vi "multicolumn_pass.vi"(0 "LstBox Refnum":refnum<vi>, 1 "Frekanslar":dbl[](array[numeric]), 2 "interrupt(F)":bool, 5 "MCListbox Refnum":refnum<vi>, 7 "Denge Kosulu x2_y2":dbl[][](array[numeric]), 9 "Denge Kosulu x1_x2":dbl[][](array[numeric]), 11 "Denge Kosulu y1_y2":dbl[][](array[numeric]), 12 "frekans index":dbl, 13 "F values array":dbl[][](array[numeric])) -> (4 "Output Denge Kosulu x2_y2":dbl[][](array[numeric]), 6 "Output Denge Kosulu x1_x2":dbl[][](array[numeric]), 8 "Outpu Denge Kosulu y1_y2":dbl[][](array[numeric]))   [LabVIEW 2014]
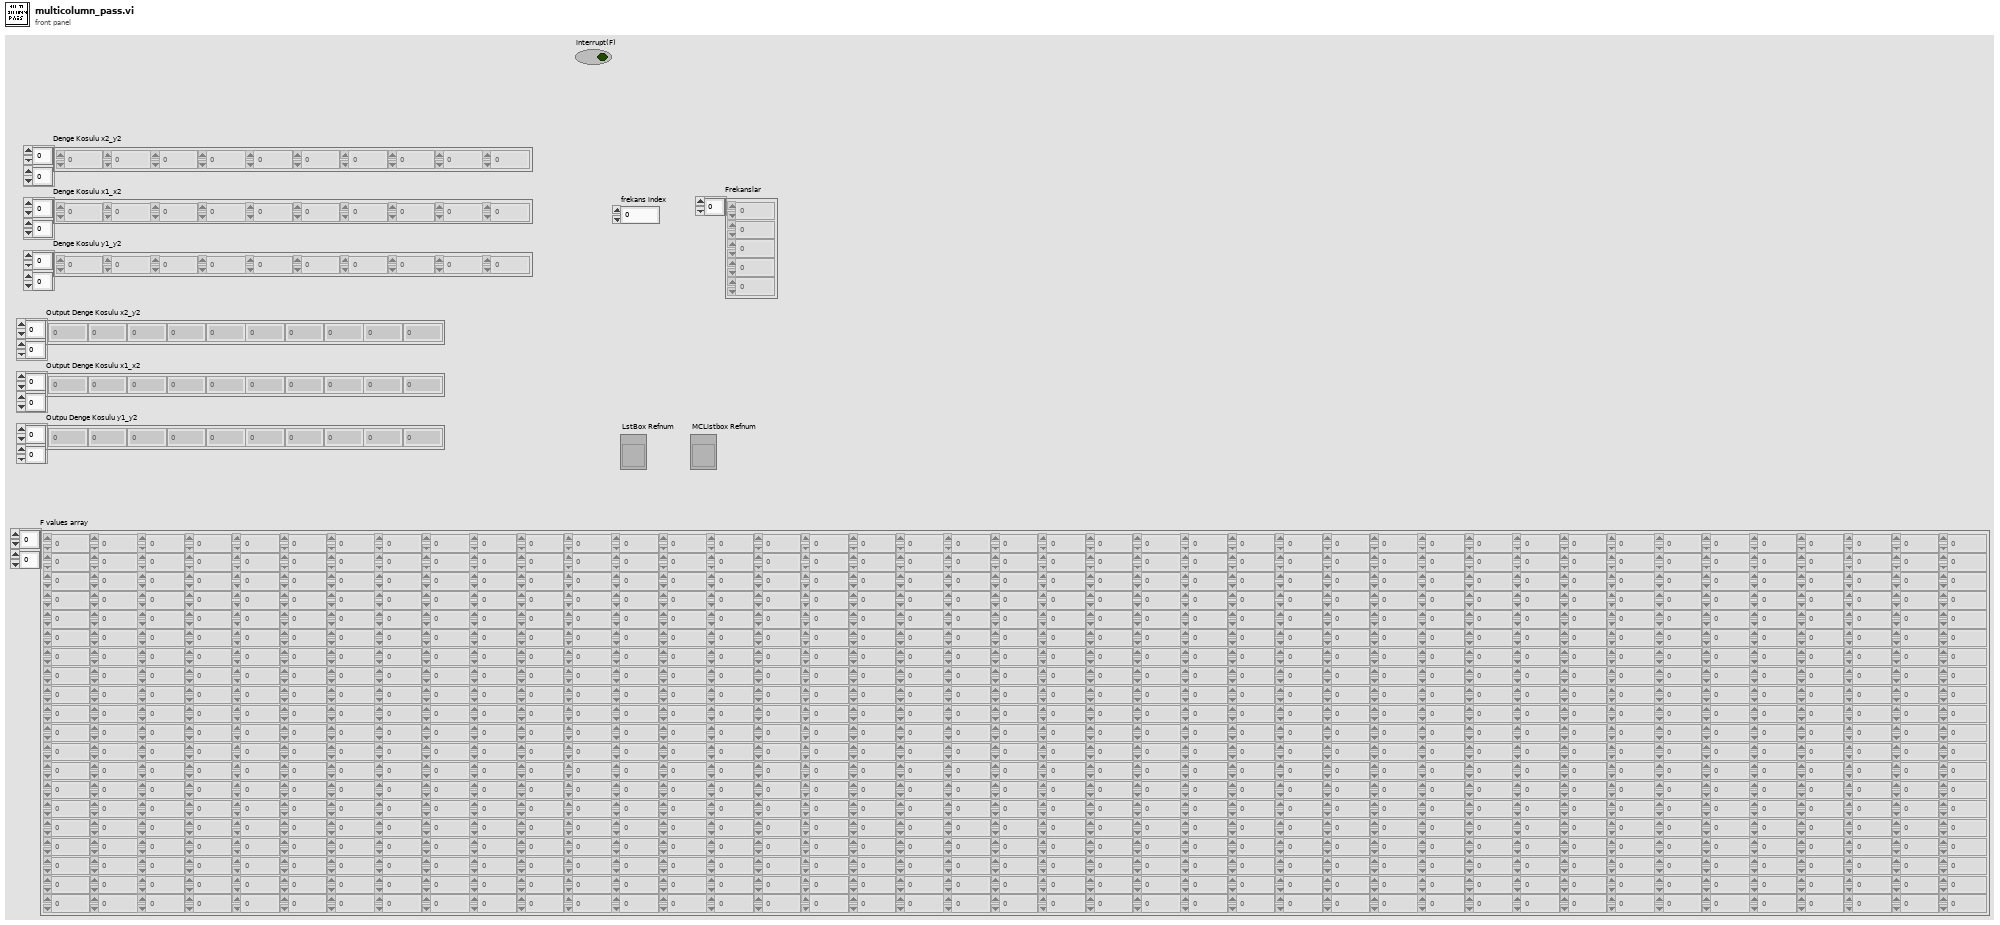
[diagram p1: front panel]
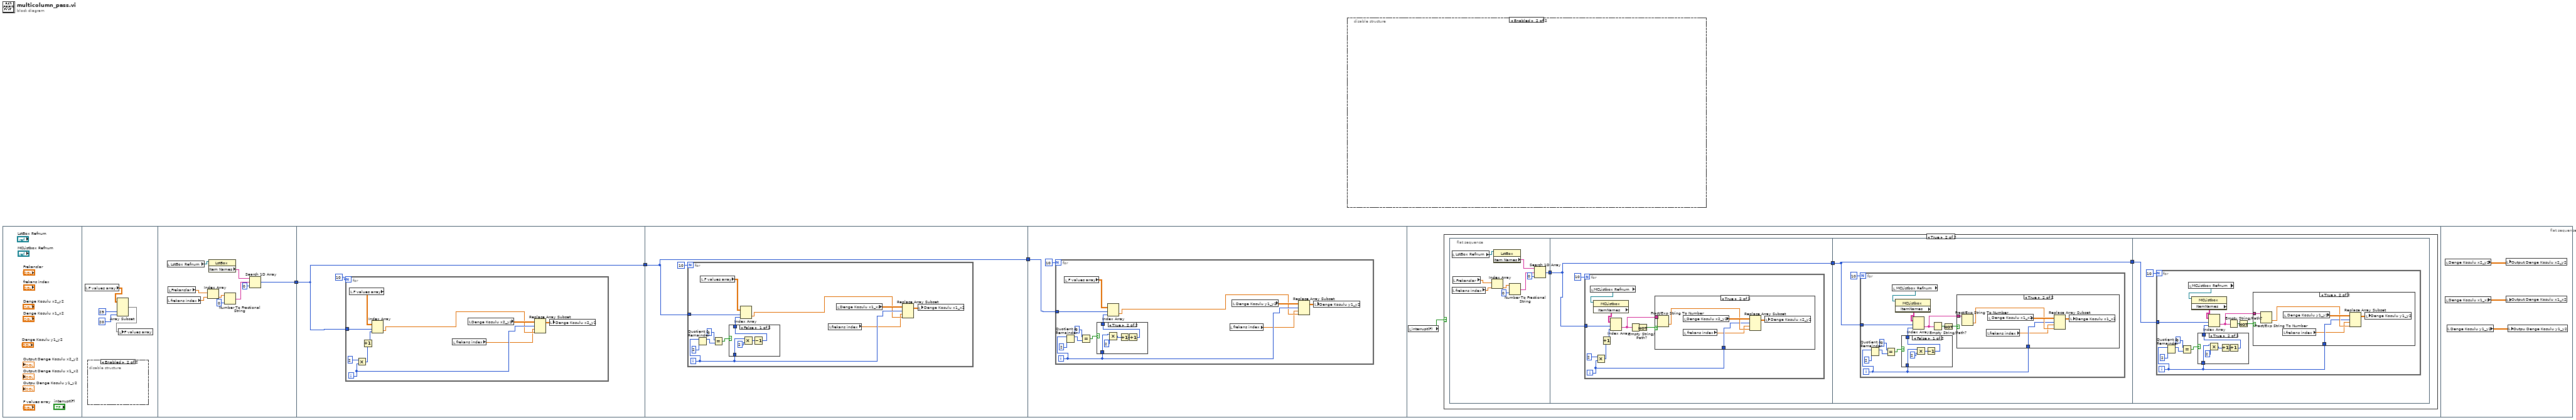
[diagram p0: block diagram]
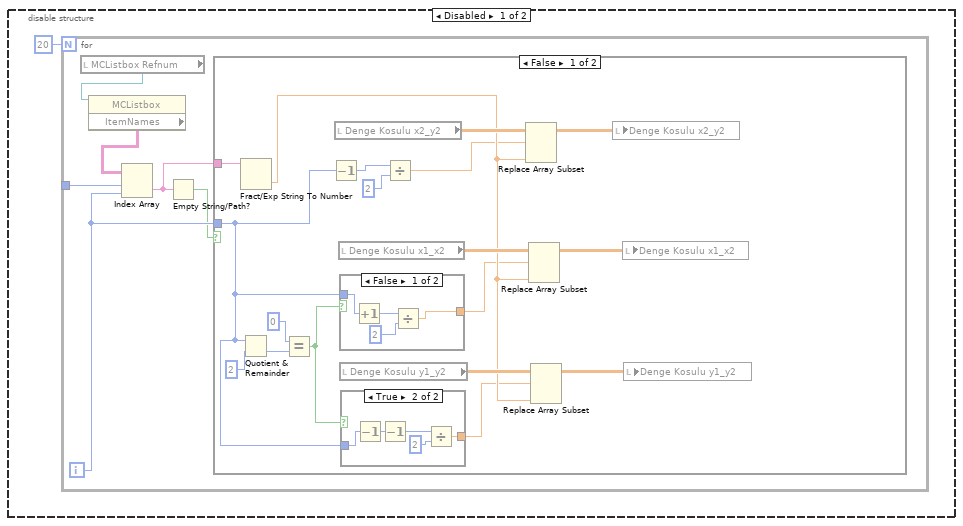
[diagram p2: hidden frame]
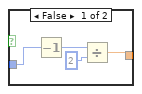
[diagram p3: hidden frame]
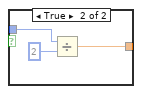
[diagram p4: hidden frame]
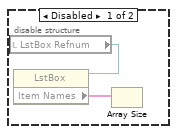
[diagram p6: hidden frame]
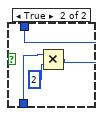
[diagram p7: hidden frame]
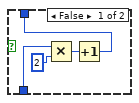
[diagram p8: hidden frame]
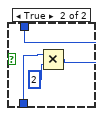
[diagram p11: hidden frame]
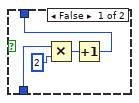
[diagram p13: hidden frame]
diagram:
  n1 = flat-sequence {
    tunnel: [w11] -> w3
    tunnel: w3 -> [w20]
    tunnel: [w20] -> w2
    tunnel: w2 -> [w32]
    tunnel: [w32] -> w1
    tunnel: w1 -> [w53]
    frame #0 {
    }
    frame #1 {
      n2 = local read "F values array"() -> (w7:dbl[][])
      n3 = disable-structure shown="Enabled" {
        frame Disabled {
          n4 = local read "LstBox Refnum"() -> (w10:refnum<vi>)
          n5 = property class="LstBox"(reference=w10) -> ("Item Names"=w9:string[])  [unwired: 1 in, 2 out]
          n6 = Array Size(array=w9) -> (size(s)=w8:i32)
        }
        frame Enabled {
        }
      }
      n7 = Array Subset(array=w7, index (col)=29 ("index"), length (col)=20 ("length")) -> (w4:dbl[][])  [unwired: 2 in]
      n8 = local write "F values array"(w4) -> ()
    }
    frame #2 {
      n9 = local read "LstBox Refnum"() -> (w19:refnum<vi>)
      n10 = local read "frekans index"() -> (w17:dbl)
      n11 = local read "Frekanslar"() -> (w18:dbl[])
      n12 = Index Array(array=w18, index=w17) -> (element=w16:dbl)
      n13 = property class="LstBox"(reference=w19) -> ("Item Names"=w15:string[])  [unwired: 1 in, 2 out]
      n14 = Number To Fractional String(number=w16, precision (6)=i16 0) -> (F-format string=w14:string)  [unwired: 2 in]
      n15 = Search 1D Array(1D array=w15, element=w14, start index (0)=0) -> (index of element=w11:i32)
    }
    frame #3 {
      n16 = for {
        N: 10 -> [_]
        tunnel: w20 -> [w27]
        i -> [w28]
        n17 = local read "F values array"() -> (w26:dbl[][])
        n18 = Multiply(x=2, y=w28) -> (x*y=w30:i32)
        n19 = Increment(x=w30) -> (x+1=w29:i32)
        n20 = Index Array(array=w26, index (row)=w27, index (col)=w29) -> (element=w23:dbl)
        n21 = local read "frekans index"() -> (w22:dbl)
        n22 = local read "Denge Kosulu x2_y2"() -> (w24:dbl[][])
        n23 = Replace Array Subset(array=w24, new element=w23, index (row)=w28, index (col)=w22) -> (w25:dbl[][])
        n24 = local write "Denge Kosulu x2_y2"(w25) -> ()
      }
    }
    frame #4 {
      n25 = for {
        N: 10 -> [_]
        tunnel: w32 -> [w40]
        i -> [w42]
        n26 = Quotient & Remainder(x=w42, y=2) -> (x-y*floor(x/y)=w39:i32)  [unwired: 1 out]
        n27 = local read "F values array"() -> (w38:dbl[][])
        n28 = Equal?(x=0, y=w39) -> (x = y?=w43:bool)
        n29 = case shown="False" w43 {
          tunnel: w42 -> [w49 w52]
          tunnel: [w46 w50] -> w41
          frame False {
            n30 = Multiply(x=w49, y=2) -> (x*y=w47:i32)
            n31 = Decrement(x=w47) -> (x-1=w46:i32)
          }
          frame True {
            n32 = Multiply(x=w52, y=2) -> (x*y=w50:i32)
          }
        }
        n33 = Index Array(array=w38, index (row)=w40, index (col)=w41) -> (element=w35:dbl)
        n34 = local read "frekans index"() -> (w34:dbl)
        n35 = local read "Denge Kosulu x1_x2"() -> (w36:dbl[][])
        n36 = Replace Array Subset(array=w36, new element=w35, index (row)=w42, index (col)=w34) -> (w37:dbl[][])
        n37 = local write "Denge Kosulu x1_x2"(w37) -> ()
      }
    }
    frame #5 {
      n38 = for {
        N: 10 -> [_]
        tunnel: w53 -> [w61]
        i -> [w63]
        n39 = local read "F values array"() -> (w59:dbl[][])
        n40 = Quotient & Remainder(x=w63, y=2) -> (x-y*floor(x/y)=w60:i32)  [unwired: 1 out]
        n41 = Equal?(x=0, y=w60) -> (x = y?=w64:bool)
        n42 = case shown="True" w64 {
          tunnel: w63 -> [w70 w75]
          tunnel: [w67 w71] -> w62
          frame False {
            n43 = Multiply(x=w70, y=2) -> (x*y=w68:i32)
            n44 = Increment(x=w68) -> (x+1=w67:i32)
          }
          frame True {
            n45 = Multiply(x=w75, y=2) -> (x*y=w73:i32)
            n46 = Increment(x=w73) -> (x+1=w72:i32)
            n47 = Increment(x=w72) -> (x+1=w71:i32)
          }
        }
        n48 = Index Array(array=w59, index (row)=w61, index (col)=w62) -> (element=w56:dbl)
        n49 = local read "frekans index"() -> (w55:dbl)
        n50 = local read "Denge Kosulu y1_y2"() -> (w57:dbl[][])
        n51 = Replace Array Subset(array=w57, new element=w56, index (row)=w63, index (col)=w55) -> (w58:dbl[][])
        n52 = local write "Denge Kosulu y1_y2"(w58) -> ()
      }
    }
    frame #6 {
      n53 = local read "interrupt(F)"() -> (w76:bool)
      n54 = case shown="True" w76 {
        frame False {
        }
        frame True {
          n55 = flat-sequence {
            tunnel: [w88] -> w79
            tunnel: w79 -> [w89]
            tunnel: [w89] -> w78
            tunnel: w78 -> [w107]
            tunnel: [w107] -> w77
            tunnel: w77 -> [w134]
            frame #0 {
              n56 = local read "LstBox Refnum"() -> (w87:refnum<vi>)
              n57 = local read "frekans index"() -> (w85:dbl)
              n58 = local read "Frekanslar"() -> (w86:dbl[])
              n59 = Index Array(array=w86, index=w85) -> (element=w84:dbl)
              n60 = property class="LstBox"(reference=w87) -> ("Item Names"=w83:string[])  [unwired: 1 in, 2 out]
              n61 = Number To Fractional String(number=w84, precision (6)=i16 0) -> (F-format string=w82:string)  [unwired: 2 in]
              n62 = Search 1D Array(1D array=w83, element=w82, start index (0)=0) -> (index of element=w88:i32)
            }
            frame #1 {
              n63 = for {
                N: 10 -> [_]
                tunnel: w89 -> [w92]
                i -> [w93]
                n64 = local read "MCListbox Refnum"() -> (w100:refnum<vi>)
                n65 = property class="MCListbox"(reference=w100) -> ("ItemNames"=w99:string[][])  [unwired: 1 in, 2 out]
                n66 = Multiply(x=2, y=w93) -> (x*y=w97:i32)
                n67 = Increment(x=w97) -> (x+1=w96:i32)
                n68 = Index Array(array=w99, index (row)=w92, index (col)=w96) -> (element=w94:string)
                n69 = Empty String/Path?(string/path=w94) -> (empty?=w95:bool)
                n70 = Not(x=w95) -> (.not. x?=w91:bool)
                n71 = case shown="True" w91 {
                  tunnel: w94 -> [_ w106]
                  tunnel: w93 -> [_ w102]
                  frame False {
                  }
                  frame True {
                    n72 = Fract/Exp String To Number(string=w106) -> (number=w103:dbl)  [unwired: 3 in, 1 out]
                    n73 = local read "Denge Kosulu x2_y2"() -> (w104:dbl[][])
                    n74 = local read "frekans index"() -> (w101:dbl)
                    n75 = Replace Array Subset(array=w104, new element=w103, index (row)=w102, index (col)=w101) -> (w105:dbl[][])
                    n76 = local write "Denge Kosulu x2_y2"(w105) -> ()
                  }
                }
              }
            }
            frame #2 {
              n77 = for {
                N: 10 -> [_]
                tunnel: w107 -> [w111]
                i -> [w113]
                n78 = Quotient & Remainder(x=w113, y=2) -> (x-y*floor(x/y)=w109:i32)  [unwired: 1 out]
                n79 = Equal?(x=0, y=w109) -> (x = y?=w114:bool)
                n80 = local read "MCListbox Refnum"() -> (w120:refnum<vi>)
                n81 = property class="MCListbox"(reference=w120) -> ("ItemNames"=w119:string[][])  [unwired: 1 in, 2 out]
                n82 = case shown="False" w114 {
                  tunnel: w113 -> [w124 w127]
                  tunnel: [w121 w125] -> w112
                  frame False {
                    n83 = Multiply(x=w124, y=2) -> (x*y=w122:i32)
                    n84 = Decrement(x=w122) -> (x-1=w121:i32)
                  }
                  frame True {
                    n85 = Multiply(x=w127, y=2) -> (x*y=w125:i32)
                  }
                }
                n86 = Index Array(array=w119, index (row)=w111, index (col)=w112) -> (element=w117:string)
                n87 = Empty String/Path?(string/path=w117) -> (empty?=w118:bool)
                n88 = Not(x=w118) -> (.not. x?=w110:bool)
                n89 = case shown="True" w110 {
                  tunnel: w117 -> [_ w133]
                  tunnel: w113 -> [_ w129]
                  frame False {
                  }
                  frame True {
                    n90 = Fract/Exp String To Number(string=w133) -> (number=w130:dbl)  [unwired: 3 in, 1 out]
                    n91 = local read "frekans index"() -> (w128:dbl)
                    n92 = local read "Denge Kosulu x1_x2"() -> (w131:dbl[][])
                    n93 = Replace Array Subset(array=w131, new element=w130, index (row)=w129, index (col)=w128) -> (w132:dbl[][])
                    n94 = local write "Denge Kosulu x1_x2"(w132) -> ()
                  }
                }
              }
            }
            frame #3 {
              n95 = for {
                N: 10 -> [_]
                tunnel: w134 -> [w138]
                i -> [w140]
                n96 = Quotient & Remainder(x=w140, y=2) -> (x-y*floor(x/y)=w136:i32)  [unwired: 1 out]
                n97 = Equal?(x=0, y=w136) -> (x = y?=w141:bool)
                n98 = local read "MCListbox Refnum"() -> (w147:refnum<vi>)
                n99 = property class="MCListbox"(reference=w147) -> ("ItemNames"=w146:string[][])  [unwired: 1 in, 2 out]
                n100 = case shown="True" w141 {
                  tunnel: w140 -> [w151 w156]
                  tunnel: [w148 w152] -> w139
                  frame False {
                    n101 = Multiply(x=w151, y=2) -> (x*y=w149:i32)
                    n102 = Increment(x=w149) -> (x+1=w148:i32)
                  }
                  frame True {
                    n103 = Multiply(x=w156, y=2) -> (x*y=w154:i32)
                    n104 = Increment(x=w154) -> (x+1=w153:i32)
                    n105 = Increment(x=w153) -> (x+1=w152:i32)
                  }
                }
                n106 = Index Array(array=w146, index (row)=w138, index (col)=w139) -> (element=w144:string)
                n107 = Empty String/Path?(string/path=w144) -> (empty?=w145:bool)
                n108 = Not(x=w145) -> (.not. x?=w137:bool)
                n109 = case shown="True" w137 {
                  tunnel: w144 -> [_ w162]
                  tunnel: w140 -> [_ w158]
                  frame False {
                  }
                  frame True {
                    n110 = Fract/Exp String To Number(string=w162) -> (number=w159:dbl)  [unwired: 3 in, 1 out]
                    n111 = local read "frekans index"() -> (w157:dbl)
                    n112 = local read "Denge Kosulu y1_y2"() -> (w160:dbl[][])
                    n113 = Replace Array Subset(array=w160, new element=w159, index (row)=w158, index (col)=w157) -> (w161:dbl[][])
                    n114 = local write "Denge Kosulu y1_y2"(w161) -> ()
                  }
                }
              }
            }
          }
        }
      }
    }
    frame #7 {
      n115 = local read "Denge Kosulu x2_y2"() -> (w165:dbl[][])
      n116 = local read "Denge Kosulu x1_x2"() -> (w164:dbl[][])
      n117 = local read "Denge Kosulu y1_y2"() -> (w163:dbl[][])
      n118 = local write "Output Denge Kosulu x2_y2"(w165) -> ()
      n119 = local write "Output Denge Kosulu x1_x2"(w164) -> ()
      n120 = local write "Outpu Denge Kosulu y1_y2"(w163) -> ()
    }
  }
  n121 = disable-structure shown="Enabled" {
    frame Disabled {
      n122 = for {
        N: 20 -> [_]
        tunnel: [w171] -> w167
        i -> [w169]
        n123 = local read "MCListbox Refnum"() -> (w173:refnum<vi>)
        n124 = property class="MCListbox"(reference=w173) -> ("ItemNames"=w172:string[][])  [unwired: 1 in, 2 out]
        n125 = Index Array(array=w172, index (row)=w171, index (col)=w169) -> (element=w170:string)
        n126 = Empty String/Path?(string/path=w170) -> (empty?=w168:bool)
        n127 = case shown="False" w168 {
          tunnel: w170 -> [w191 _]
          tunnel: w169 -> [w175 _]
          frame False {
            n128 = Fract/Exp String To Number(string=w191) -> (number=w184:dbl)  [unwired: 3 in, 1 out]
            n129 = Quotient & Remainder(x=w175, y=2) -> (floor(x/y)=w179:i32)  [unwired: 1 out]
            n130 = Equal?(x=0, y=w179) -> (x = y?=w177:bool)
            n131 = Decrement(x=w175) -> (x-1=w183:i32)
            n132 = local read "Denge Kosulu x2_y2"() -> (w190:dbl[][])
            n133 = local read "Denge Kosulu x1_x2"() -> (w189:dbl[][])
            n134 = case shown="False" w177 {
              tunnel: w175 -> [w204 w207]
              tunnel: [w201 w205] -> w176
              frame False {
                n135 = Increment(x=w204) -> (x+1=w203:i32)
                n136 = Divide(x=w203, y=2) -> (x/y=w201:dbl)
              }
              frame True {
                n137 = Divide(x=w207, y=2) -> (x/y=w205:dbl)
              }
            }
            n138 = local read "Denge Kosulu y1_y2"() -> (w188:dbl[][])
            n139 = case shown="True" w177 {
              tunnel: w175 -> [w193 w200]
              tunnel: [w192 w196] -> w174
              frame False {
                n140 = Decrement(x=w193) -> (x-1=w195:i32)
                n141 = Divide(x=w195, y=2) -> (x/y=w192:dbl)
              }
              frame True {
                n142 = Decrement(x=w200) -> (x-1=w199:i32)
                n143 = Decrement(x=w199) -> (x-1=w198:i32)
                n144 = Divide(x=w198, y=2) -> (x/y=w196:dbl)
              }
            }
            n145 = Divide(x=w183, y=2) -> (x/y=w181:dbl)
            n146 = Replace Array Subset(array=w190, new element=w184, index (row)=w181) -> (w187:dbl[][])  [unwired: 1 in]
            n147 = Replace Array Subset(array=w189, new element=w184, index (row)=w176) -> (w186:dbl[][])  [unwired: 1 in]
            n148 = Replace Array Subset(array=w188, new element=w184, index (row)=w174) -> (w185:dbl[][])  [unwired: 1 in]
            n149 = local write "Denge Kosulu x2_y2"(w187) -> ()
            n150 = local write "Denge Kosulu x1_x2"(w186) -> ()
            n151 = local write "Denge Kosulu y1_y2"(w185) -> ()
          }
          frame True {
          }
        }
      }
    }
    frame Enabled {
    }
  }
